vi "PiezoRamp.vi"() -> ()   [LabVIEW 2015]
uses:
  <vilib>/Analysis/baseanly.llb/Mean (DBL).vi
  <vilib>/DAQmx/write.llb/DAQmx Write (Analog 1D DBL NChan 1Samp).vi
  <vilib>/DAQmx/miscellaneous.llb/DAQmx Fill In Error Info.vi
  <vilib>/Analysis/NI_AALBase.lvlib
panel:
  out "relative seconds":dbl format="%_19f"
  out "is late?":bool
  in  "timeout (s)":dbl=-1.0 format="%#_15g"
  in  "AOTF3":dbl
  in  "AOTF2":dbl
  in  "AOTF1":dbl
  in  "Zmax":dbl
  in  "Zmin":dbl
  in  "Delta Z":dbl
  in  "stop":bool
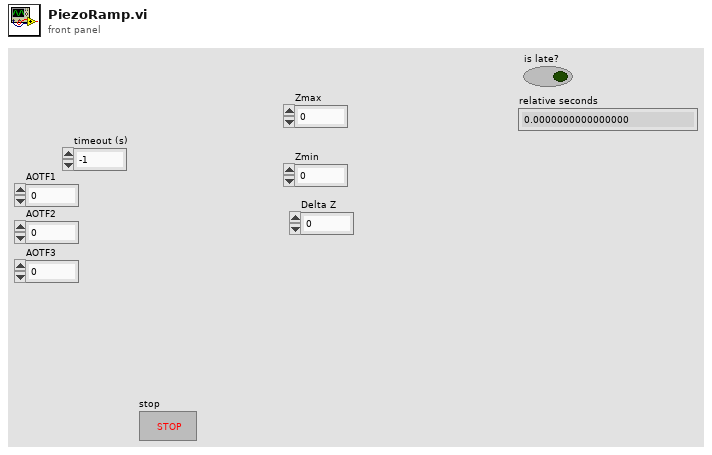
[diagram p1: front panel]
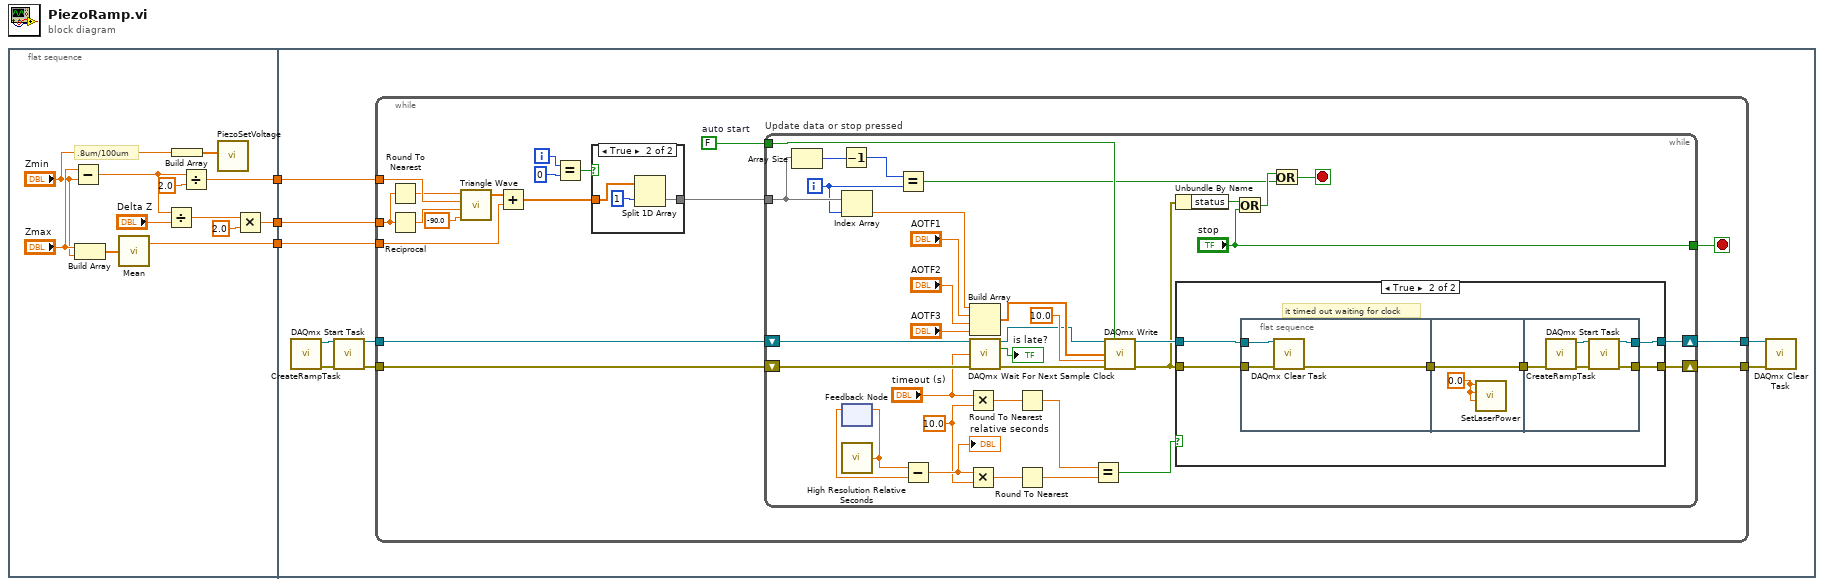
[diagram p0: block diagram]
diagram:
  n1 = flat-sequence {
    tunnel: [w6] -> w3
    tunnel: [w4] -> w2
    tunnel: [w5] -> w1
    tunnel: w3 -> [w24]
    tunnel: w2 -> [w22]
    tunnel: w1 -> [w23]
    frame #0 {
      # ".8um/100um"
      n2 = Subtract(x="Zmax", y="Zmin") -> (x-y=w14:dbl)
      n3 = Build Array("Zmax", "Zmin") -> (w9:dbl[])
      n4 = call-poly <vilib>:"Mean.vi"("X"=w9) -> ("mean"=w4:dbl)  [unwired: 1 out]
      n5 = Divide(x=w14, y="Delta Z") -> (x/y=w12:dbl)
      n6 = Build Array("Zmin") -> (w8:dbl[])
      n7 = Divide(x=w14, y=2.0) -> (x/y=w6:dbl)
      n8 = call "PiezoSetVoltage.vi"("data"=w8) -> ()  [unwired: 10 in, 1 out]
      n9 = Multiply(x=w12, y=2.0) -> (x*y=w5:dbl)
    }
    frame #1 {
      n10 = call "CreateRampTask.vi"() -> ("error out"=w18:errorcluster, "task out"=w19:refnum<k21>)  [unwired: 10 in]
      n11 = call <vilib>:"DAQmx Start Task.vi"("task/channels in"=w19, "error in"=w18) -> ("task out"=w17:refnum<k21>, "error out"=w16:errorcluster)  [unwired: 12 in]
      n12 = while {
        tunnel: w24 -> [w39]
        tunnel: w23 -> [w36]
        tunnel: w22 -> [w38]
        tunnel: [w33] -> w21
        tunnel: [w32] -> w20
        tunnel: w17 -> [w25]
        tunnel: w16 -> [w31]
        i -> [w29]
        stop <- w34 stop-if-true
        w42 = FALSE  # auto start
        n13 = Round To Nearest(number=w36) -> (nearest integer value=w37:dbl)
        n14 = Reciprocal(x=w36) -> (1/x=w35:dbl)
        n15 = call <vilib>:"Triangle Wave.vi"("samples"=w37, "amplitude"=w39, "frequency"=w35, "phase in"=-90.0) -> ("triangle wave"=w40:dbl[])  [unwired: 1 in, 2 out]
        n16 = Add(x=w40, y=w38) -> (x+y=w28:dbl[])
        n17 = Equal?(x=w29, y=0) -> (x = y?=w30:bool)
        n18 = case shown="True" w30 {
          tunnel: w28 -> [w43 w46]
          tunnel: [w43 w45] -> w27
          frame False {
          }
          frame True {
            n19 = Split 1D Array(array=w46, index=1) -> (second subarray=w45:dbl[])  [unwired: 1 out]
          }
        }
        n20 = while "Update data or stop pressed" {
          tunnel: w42 -> [w80]
          shift-right: [w51] -> w33
          shift-left: w31 -> [w68]
          tunnel: w27 -> [w72]
          tunnel: ["stop"] -> w34
          shift-right: [w50] -> w32
          shift-left: w25 -> [w49]
          i -> [w71]
          stop <- w77 stop-if-true
          w59 = 10.0 ("y")
          n21 = Array Size(array=w72) -> (size(s)=w76:i32)
          n22 = Decrement(x=w76) -> (x-1=w75:i32)
          n23 = Index Array(array=w72, index=w71) -> (element=w70:dbl)
          n24 = feedback #1() -> (w61:dbl)  [unwired: 1 in]
          n25 = call <vilib>:"High Resolution Relative Seconds.vi"() -> ("relative seconds"=w62:dbl)
          n26 = feedback-in #1(w62) -> ()
          n27 = Equal?(x=w75, y=w71) -> (x = y?=w74:bool)
          n28 = Subtract(x=w62, y=w61) -> (x-y=w60:dbl)
          "relative seconds" <- w60
          n29 = Multiply(x="timeout (s)", y=w59) -> (x*y=w57:dbl)
          n30 = Multiply(x=w60, y=w59) -> (x*y=w56:dbl)
          n31 = Build Array(w70, "AOTF1", "AOTF2", "AOTF3") -> (w69:dbl[])
          n32 = call <vilib>:"DAQmx Wait For Next Sample Clock.vi"("task/channels in"=w49, "timeout (sec)"="timeout (s)", "error in"=w68) -> ("task out"=w67:refnum<k21>, "is late?"=→"is late?":bool, "error out"=w47:errorcluster)  [unwired: 10 in]
          n33 = Round To Nearest(number=w57) -> (nearest integer value=w55:dbl)
          n34 = Round To Nearest(number=w56) -> (nearest integer value=w54:dbl)
          n35 = Equal?(x=w55, y=w54) -> (x = y?=w48:bool)
          n36 = call-poly <vilib>:"DAQmx Write.vi"("task/channels in"=w67, "auto start"=w80, "data"=w69, "timeout"=10.0, "error in"=w47) -> ("task out"=w53:refnum<k21>, "error out"=w52:errorcluster)  [unwired: 8 in, 1 out]
          n37 = Unbundle By Name(w52) -> ("status"=w81:bool)
          n38 = case shown="True" w48 {
            tunnel: w53 -> [w82 w89]
            tunnel: [w83 w86] -> w51
            tunnel: w52 -> [w83 w88]
            tunnel: [w82 w87] -> w50
            frame False {
            }
            frame True {
              # "it timed out waiting for clock"
              n39 = flat-sequence {
                tunnel: w89 -> [w92]
                tunnel: w88 -> [w91]
                tunnel: [w90] -> w84
                tunnel: [w93] -> w85
                tunnel: w84 -> [w93]
                tunnel: [w97] -> w87
                tunnel: [w96] -> w86
                tunnel: w85 -> [w95]
                frame #0 {
                  n40 = call <vilib>:"DAQmx Clear Task.vi"("task in"=w92, "error in"=w91) -> ("error out"=w90:errorcluster)  [unwired: 13 in]
                }
                frame #1 {
                  w94 = 0.0 ("AOTF1")
                  n41 = call "SetLaserPower.vi"("AOTF3"=w94, "AOTF2"=w94, "AOTF1"=w94) -> ()  [unwired: 8 in, 1 out]
                }
                frame #2 {
                  n42 = call "CreateRampTask.vi"("error in"=w95) -> ("error out"=w99:errorcluster, "task out"=w98:refnum<k21>)  [unwired: 9 in]
                  n43 = call <vilib>:"DAQmx Start Task.vi"("task/channels in"=w98, "error in"=w99) -> ("task out"=w97:refnum<k21>, "error out"=w96:errorcluster)  [unwired: 12 in]
                }
              }
            }
          }
          n44 = Or(x=w81, y="stop") -> (x .or. y?=w78:bool)
          n45 = Or(x=w78, y=w74) -> (x .or. y?=w77:bool)
        }
      }
      n46 = call <vilib>:"DAQmx Clear Task.vi"("task in"=w20, "error in"=w21) -> ()  [unwired: 13 in, 1 out]
    }
  }
